vi "Validate Column Names.vi"(8 "error in (no error)":errorcluster, 11 "Label.Text":string) -> (0 "error out":errorcluster, 3 "result string":string)   [LabVIEW 2018]
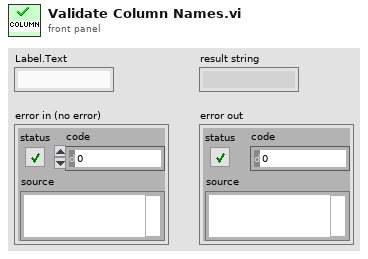
[diagram p1: front panel]
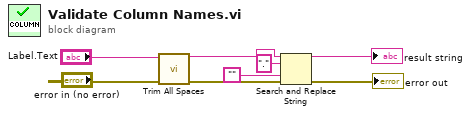
[diagram p0: block diagram]
diagram:
  n1 = call "Trim All Spaces.vi"("error in (no error)"="error in (no error)", "Label.Text"="Label.Text") -> ("error out"=w3:errorcluster, "result string"=w1:string)  [unwired: 8 in]
  n2 = Search and Replace String(input string=w1, search string=".", replace string="", error in=w3) -> (result string=→"result string":string, error out=→"error out":errorcluster)  [unwired: 4 in, 2 out]
